vi "salidas_Muestreo_continuo.vi"() -> ()   [LabVIEW 2021]
uses:
  <vilib>/DAQmx/write.llb/DAQmx Write (Analog 2D DBL NChan NSamp).vi
  <vilib>/DAQmx/create/channels.llb/DAQmx Create Channel (AO-Voltage-Basic).vi
  <vilib>/DAQmx/configure/timing.llb/DAQmx Timing (Sample Clock).vi
  <vilib>/DAQmx/miscellaneous.llb/DAQmx Fill In Error Info.vi
panel:
  out "XY Graph":cluster{dbl[], dbl[]}(graph)
  out "Waveform Graph":dbl[][](graph)
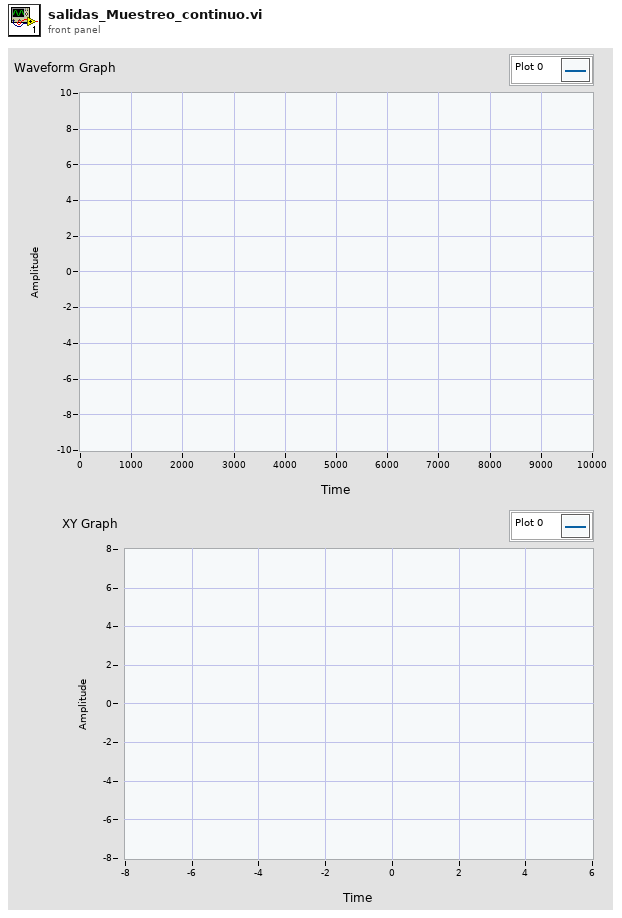
[diagram p1: front panel]
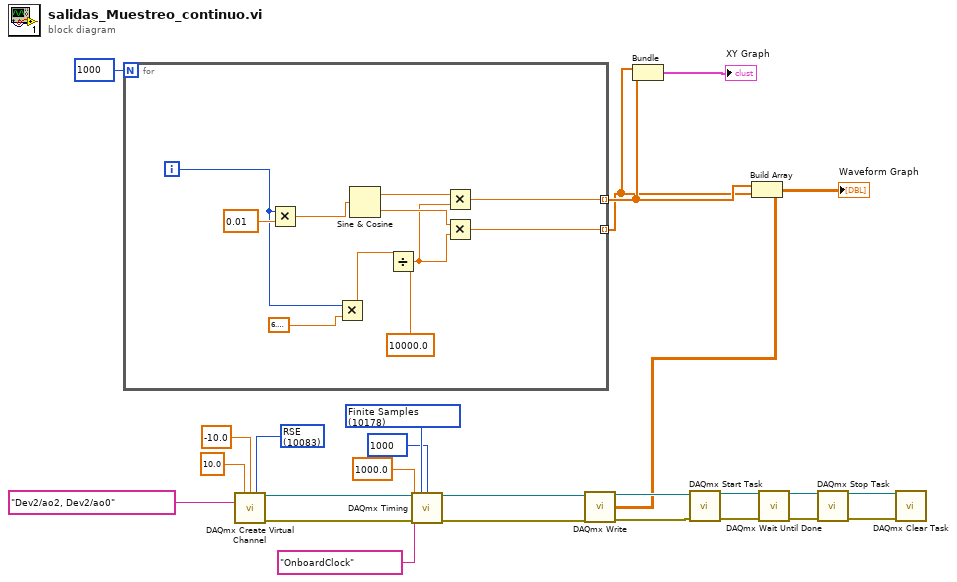
[diagram p0: block diagram]
diagram:
  w4 = 10178 items=["Finite Samples"=10178, "Continuous Samples"=10123, "Hardware Timed Single Point"=12522] ("sample mode")
  w7 = 10083 items=["Default"=-1, "RSE"=10083, "Differential"=10106, "Pseudodifferential"=12529] ("output terminal configuration")
  n1 = for {
    N: 1000 -> [_]
    tunnel: [w32] -> w23 mode=indexing
    tunnel: [w31] -> w2 mode=indexing
    i -> [w30]
    n2 = Multiply(x=w30, y=0.01) -> (x*y=w35:dbl)
    n3 = Multiply(x=w30, y=6.283185307179586) -> (x*y=w27:dbl)
    n4 = Sine & Cosine(0:w35) -> (1:w34:dbl, 2:w33:dbl)
    n5 = Divide(x=w27, y=10000.0 ("x")) -> (x/y=w28:dbl)
    n6 = Multiply(x=w34, y=w28) -> (x*y=w32:dbl)
    n7 = Multiply(x=w33, y=w28) -> (x*y=w31:dbl)
  }
  n8 = call-poly <vilib>:"DAQmx Create Virtual Channel.vi"("maximum value"=10.0, "minimum value"=-10.0, "output terminal configuration"=w7, "physical channels"=tag "Dev2/ao2, Dev2/ao0") -> ("task out"=w15:refnum<k21>, "error out"=w16:errorcluster)  [unwired: 10 in]
  n9 = call-poly <vilib>:"DAQmx Timing.vi"("task/channels in"=w15, "sample mode"=w4, "samples per channel"=1000, "rate"=1000.0, "source"=tag "OnboardClock", "error in"=w16) -> ("task out"=w14:refnum<k21>, "error out"=w13:errorcluster)  [unwired: 8 in]
  n10 = Bundle(w2, w23) -> (→"XY Graph":cluster{dbl[], dbl[]})  [unwired: 1 in]
  n11 = Build Array(w23, w2) -> (w1:dbl[][])
  "Waveform Graph" <- w1
  n12 = call-poly <vilib>:"DAQmx Write.vi"("task/channels in"=w14, "data"=w1, "error in"=w13) -> ("task out"=w12:refnum<k21>, "error out"=w11:errorcluster)  [unwired: 10 in, 1 out]
  n13 = call <vilib>:"DAQmx Start Task.vi"("task/channels in"=w12, "error in"=w11) -> ("task out"=w22:refnum<k21>, "error out"=w19:errorcluster)  [unwired: 12 in]
  n14 = call <vilib>:"DAQmx Wait Until Done.vi"("task/channels in"=w22, "error in"=w19) -> ("task out"=w21:refnum<k21>, "error out"=w18:errorcluster)  [unwired: 12 in]
  n15 = call <vilib>:"DAQmx Stop Task.vi"("task/channels in"=w21, "error in"=w18) -> ("task out"=w20:refnum<k21>, "error out"=w17:errorcluster)  [unwired: 12 in]
  n16 = call <vilib>:"DAQmx Clear Task.vi"("task in"=w20, "error in"=w17) -> ()  [unwired: 13 in, 1 out]
